vi "CgInfo.vi"(0 "VISA resource name":refnum<visa-resource-name>="COM1", 11 "error in (no error)":errorcluster) -> (4 "VISA resource name out":refnum<visa-resource-name>, 6 "#Sensors":i32, 10 "RH?":bool, 12 "Sensor Names":string[](array[string]), 13 "Sensors Active":bool[](array[boolean]), 14 "Hardware Calibration":u8[][](array[numeric]), 15 "error out":errorcluster)   [LabVIEW 2012]
doc: "Queries the cyberglove and returns data about its current settings and state including:\nThe handedness of the glove\nHow many and which sensors are currently active.\n\nSpecific Outputs:\nRH?: True if glove is right-handed\nSensors active: a binary array of which sensors (of the list of 24 from the manual) output data\nSensor Names: the names of the sensors producing data (which joint they correspond to)s"
uses:
  <vilib>/Instr/_visa.llb/VISA Configure Serial Port (Instr).vi
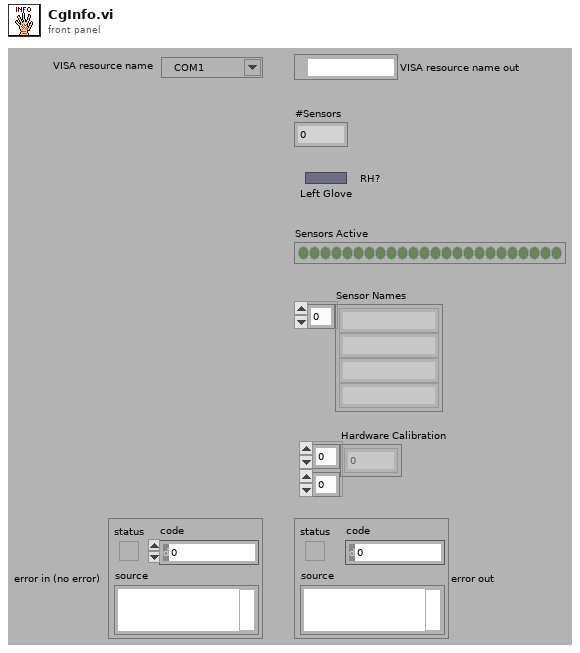
[diagram p1: front panel]
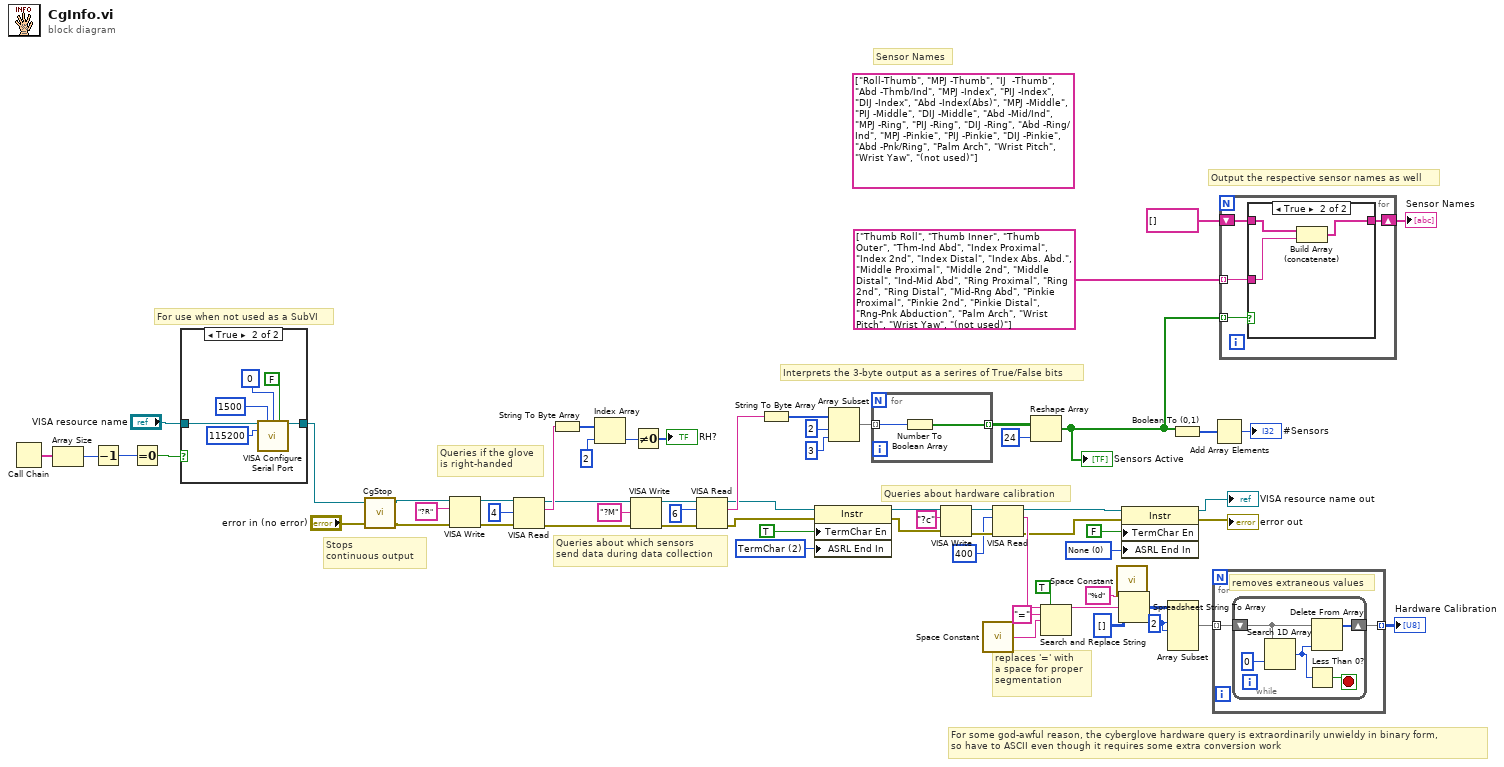
[diagram p0: block diagram]
diagram:
  w3 = u16 0 items=["None", "Last Bit", "TermChar"] ("Serial Settings:End Mode for Reads")
  w16 = u16 2 items=["None", "Last Bit", "TermChar"] ("Serial Settings:End Mode for Reads")
  w25 = 2 ("index")
  (unwired) string[] ["Roll-Thumb", "MPJ -Thumb", "IJ  -Thumb", "Abd -Thmb/Ind", "MPJ -Index", "PIJ -Index", "DIJ -Index", "Abd -Index(Abs)", "MPJ -Middle", "PIJ -Middle", "DIJ -Middle", "Abd -Mid/Ind", "MPJ -Ring", "PIJ -Ring", "DIJ -Ring", "Abd -Ring/Ind", "MPJ -Pinkie", "PIJ -Pinkie", "DIJ -Pinkie", "Abd -Pnk/Ring", "Palm Arch", "Wrist Pitch", "Wrist Yaw", "(not used)"]
  # "Queries about hardware calibration"
  # "replaces '=' with\na space for proper\nsegmentation"
  # "For some god-awful reason, the cyberglove hardware query is extraordinarily unwieldy in binary form,\nso have to ASCII even though it requires some extra conversion work"
  # "Output the respective sensor names as well"
  # "Interprets the 3-byte output as a serires of True/False bits"
  # "Queries about which sensors \nsend data during data collection"
  # "Queries if the glove\nis right-handed"
  # "Sensor Names"
  # "Stops \ncontinuous output"
  # "For use when not used as a SubVI"
  n1 = Call Chain() -> (call chain=w42:string[])
  n2 = Array Size(array=w42) -> (size(s)=w41:i32)
  n3 = Decrement(x=w41) -> (x-1=w40:i32)
  n4 = Equal To 0?(x=w40) -> (x = 0?=w39:bool)
  n5 = case shown="True" w39 {
    tunnel: "VISA resource name" -> [w66 w72]
    tunnel: [w66 w71] -> w31
    frame False {
    }
    frame True {
      n6 = call-poly "VISA Configure Serial Port"("VISA resource name"=w72, "timeout (10sec)"=u32 1500, "termination char\n(0xA = '\\n' = LF)"=u8 0 ("termination char\n(0xA = '\\n' = LF)"), "Enable Termination\nChar (T)"=FALSE ("Enable Termination\nChar (T)"), "baud rate (9600)"=u32 115200) -> ("VISA resource name out"=w71:refnum<visa-resource-name>)  [unwired: 9 in, 1 out]
    }
  }
  n7 = call "CgStop.vi"("error in (no error)"="error in (no error)", "VISA resource name"=w31) -> ("error out"=w29:errorcluster, "VISA resource name out"=w30:refnum<visa-resource-name>)  [unwired: 2 in]
  n8 = VISA Write(VISA resource name=w30, write buffer="?R", error in (no error)=w29) -> (VISA resource name out=w63:refnum<visa-resource-name>, error out=w62:errorcluster)  [unwired: 1 out]
  n9 = VISA Read(VISA resource name=w63, byte count=u32 4, error in (no error)=w62) -> (VISA resource name out=w50:refnum<visa-resource-name>, read buffer=w60:string, error out=w51:errorcluster)  [unwired: 1 out]
  n10 = String To Byte Array(string=w60) -> (unsigned byte array=w59:u8[])
  n11 = Index Array(array=w59, index=2) -> (element=w57:u8)
  n12 = VISA Write(VISA resource name=w50, write buffer="?M", error in (no error)=w51) -> (VISA resource name out=w54:refnum<visa-resource-name>, error out=w53:errorcluster)  [unwired: 1 out]
  n13 = Not Equal To 0?(x=w57) -> (x != 0?=→"RH?":bool)
  n14 = VISA Read(VISA resource name=w54, byte count=u32 6, error in (no error)=w53) -> (VISA resource name out=w14:refnum<visa-resource-name>, read buffer=w49:string, error out=w15:errorcluster)  [unwired: 1 out]
  n15 = String To Byte Array(string=w49) -> (unsigned byte array=w48:u8[])
  n16 = property class="Instr"(reference=w14, error in=w15, "TermChar En"=TRUE ("Message Based Settings:Termination Character Enable"), "ASRL End In"=w16) -> (reference out=w2:refnum<visa-resource-name>, error out=w1:errorcluster)
  n17 = Array Subset(array=w48, index=2, length=3) -> (w45:u8[])
  n18 = for {
    tunnel: w45 -> [w74] mode=indexing
    tunnel: [w73] -> w44 mode=indexing
    n19 = Number To Boolean Array(number=w74) -> (Boolean array=w73:bool[])
  }
  n20 = VISA Write(VISA resource name=w2, write buffer="?c", error in (no error)=w1) -> (VISA resource name out=w9:refnum<visa-resource-name>, error out=w8:errorcluster)  [unwired: 1 out]
  n21 = call <vilib>:"Space Constant.vi"() -> ("String"=w20:string)
  n22 = VISA Read(VISA resource name=w9, byte count=u32 400, error in (no error)=w8) -> (VISA resource name out=w6:refnum<visa-resource-name>, read buffer=w22:string, error out=w5:errorcluster)  [unwired: 1 out]
  n23 = Reshape Array(w44, 24 ("dimension size")) -> (w36:bool[])
  "Sensors Active" <- w36
  n24 = Search and Replace String(replace all?=TRUE ("replace all? (F)"), input string=w22, search string="=", replace string=w20) -> (result string=w18:string)  [unwired: 4 in, 3 out]
  n25 = call <vilib>:"Space Constant.vi"() -> ("String"=w23:string)
  n26 = Spreadsheet String To Array(delimiter (Tab)=w23, format string="%d", spreadsheet string=w18, array type (2D Dbl)=u8[][] []) -> (array=w26:u8[][])
  n27 = property class="Instr"(reference=w6, error in=w5, "TermChar En"=FALSE ("Message Based Settings:Termination Character Enable"), "ASRL End In"=w3) -> (reference out=→"VISA resource name out":refnum<visa-resource-name>, error out=→"error out":errorcluster)
  n28 = Array Subset(array=w26, index (row)=w25, length (row)=w25) -> (w24:u8[][])  [unwired: 2 in]
  n29 = Boolean To (0,1)(Boolean=w36) -> (0, 1=w35:i16[])
  n30 = for {
    tunnel: w24 -> [w76] mode=indexing
    tunnel: [w75] -> w11 mode=indexing
    # "removes extraneous values"
    n31 = while {
      shift-right: [w77] -> w75
      shift-left: w76 -> [w78]
      stop <- w80 stop-if-true
      n32 = Search 1D Array(1D array=w78, element=u8 0) -> (index of element=w79:i32)  [unwired: 1 in]
      n33 = Less Than 0?(x=w79) -> (x < 0?=w80:bool)
      n34 = Delete From Array(array=w78, index=w79) -> (array with subset deleted=w77:u8[])  [unwired: 1 in, 1 out]
    }
  }
  "Hardware Calibration" <- w11
  n35 = Add Array Elements(numeric array=w35) -> (sum=→"#Sensors":i16)
  n36 = for {
    tunnel: w36 -> [w85] mode=indexing
    tunnel: string[] ["Thumb Roll", "Thumb Inner", "Thumb Outer", "Thm-Ind Abd", "Index Proximal", "Index 2nd", "Index Distal", "Index Abs. Abd.", "Middle Proximal", "Middle 2nd", "Middle Distal", "Ind-Mid Abd", "Ring Proximal", "Ring 2nd", "Ring Distal", "Mid-Rng Abd", "Pinkie Proximal", "Pinkie 2nd", "Pinkie Distal", "Rng-Pnk Abduction", "Palm Arch", "Wrist Pitch", "Wrist Yaw", "(not used)"] -> [w82] mode=indexing
    shift-right: [w83] -> w37
    shift-left: string[] [] -> [w84]
    n37 = case shown="True" w85 {
      tunnel: w84 -> [w86 w89]
      tunnel: [w86 w87] -> w83
      tunnel: w82 -> [_ w88]
      frame False {
      }
      frame True {
        n38 = Build Array (concatenate)(w89, w88) -> (w87:string[])
      }
    }
  }
  "Sensor Names" <- w37
